vi "Add.vi"(6 "Index [-1, last]":i32=-1, 7 "Data":string[](array[string]), 8 "error in (no error)":errorcluster, 9 "Child":refnum<class "CConfig Object.lvclass">, 11 "Composite Object in":refnum<class "CConfig Object.lvclass">) -> (0 "error out":errorcluster, 3 "Composite Object out":refnum<class "CConfig Object.lvclass">, 4 "Index":i32)   [LabVIEW 2013, in "CConfig Object.lvclass"]
doc: "Copyright 2018, Carya Automatisering, Wiebe Walstra."
uses:
  CConfig Object.lvclass
  CConfig Object.lvclass/CConfig Object.ctl
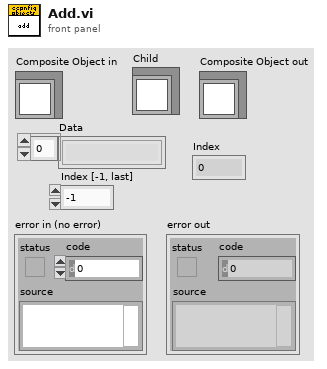
[diagram p1: front panel]
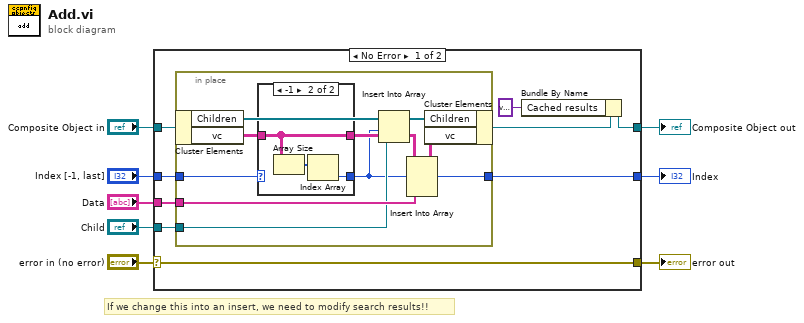
[diagram p0: block diagram]
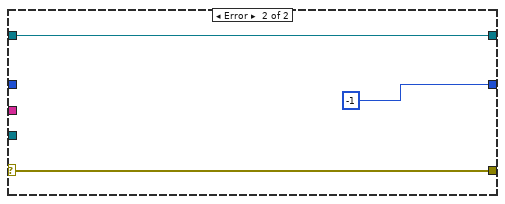
[diagram p3: hidden frame]
diagram:
  # "If we change this into an insert, we need to modify search results!!"
  n1 = case shown="No Error" "error in (no error)" {
    selector: "error in (no error)" -> [w17 w34]
    tunnel: [w17 w34] -> w7
    tunnel: [w11 w33] -> w5
    tunnel: "Composite Object in" -> [w16 w33]
    tunnel: "Data" -> [w15 _]
    tunnel: [w14 -1] -> w3
    tunnel: "Child" -> [w13 _]
    tunnel: "Index [-1, last]" -> [w9 _]
    frame No Error {
      n2 = in-place {
        in-place-border: w15 -> [w24]
        in-place-border: [w18] -> w14
        in-place-border: w13 -> [w19]
        in-place-border: w9 -> [w20]
        n3 = in-place-cluster #1(w16) -> ("Children"=w23:refnum<class>[], "vc"=w25:string[][])
        n4 = case shown="-1" w20 {
          selector: w20 -> [w27 _]
          tunnel: w25 -> [w28 w29]
          tunnel: [w27 w30] -> w18
          tunnel: [w28 w29] -> w21
          frame Default {
          }
          frame -1 {
            n5 = Array Size(array=w29) -> (size(s)=w31:i32[])
            n6 = Index Array(array=w31) -> (element=w30:i32)  [unwired: 1 in]
          }
        }
        n7 = Insert Into Array(array=w23, index=w18, new element=w19) -> (w22:refnum<class>[])
        n8 = Insert Into Array(array=w21, index (row)=w18, new element=w24) -> (w26:string[][])  [unwired: 1 in]
        n9 = in-place-cluster #1("Children"=w22, "vc"=w26) -> (w12:refnum<class "CConfig Object.lvclass">)
      }
      n10 = Bundle By Name(cluster=w12, "Cached results"=variant) -> (w11:refnum<class "CConfig Object.lvclass">)
    }
    frame Error {
    }
  }
  "error out" <- w7
  "Composite Object out" <- w5
  "Index" <- w3
